vi "StrTraining.vi"() -> ()   [LabVIEW 2015]
panel:
  out "Output-2":string
  out "NumToStrOut-1":string
  out "StrToNumOut-1":i32
  in  "Input-3":string
  out "Output-1 Len":i32
  out "Output-1":string
  in  "Input-2":string
  out "Input-1 Len":i32
  in  "Input-1":string
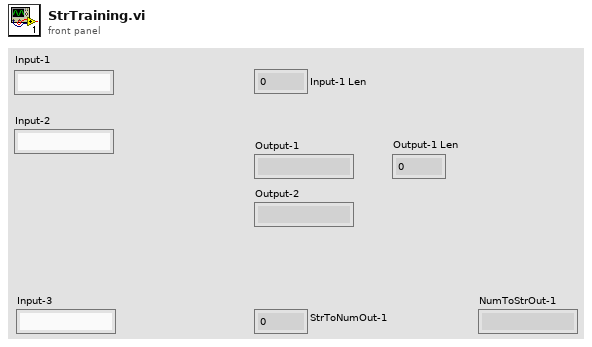
[diagram p1: front panel]
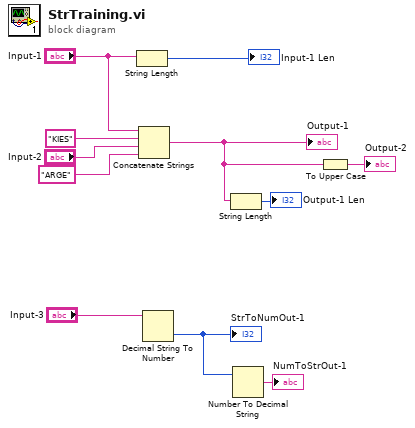
[diagram p0: block diagram]
diagram:
  n1 = String Length(string="Input-1") -> (length=→"Input-1 Len":i32)
  n2 = Concatenate Strings("Input-1", "KIES" ("string"), "Input-2", "ARGE" ("string")) -> (w1:string)
  "Output-1" <- w1
  n3 = Decimal String To Number(string="Input-3") -> (number=w4:i32)  [unwired: 2 in, 1 out]
  "StrToNumOut-1" <- w4
  n4 = String Length(string=w1) -> (length=→"Output-1 Len":i32)
  n5 = Number To Decimal String(number=w4) -> (decimal integer string=→"NumToStrOut-1":string)  [unwired: 1 in]
  n6 = To Upper Case(1:w1) -> (0:→"Output-2":string)
